vi "170519018PROJEkapalicevrimkontrolu.vi"() -> ()   [LabVIEW 2020]
uses:
  <vilib>/Instr/_visa.llb/VISA Configure Serial Port (Instr).vi
panel:
  out "ENCODER":string
  in  "PORT COM":refnum<visa-resource-name>
  in  "stop":bool
  out "PWM":i16(slide) scale=-255.0..255.0
  out "AYAR NOKTASI VE POZISYONLARI":cluster{i16, i16}(knob)={0, 73} scale=0.0..360.0
  in  "AYAR NOKTASI":i16(knob) scale=0.0..360.0
  out "GRAFIK PWM":i32(graph)
  out "GRAFIGIN AYAR NOKTASI  ve EKSEN KONUMU":cluster{"SETPOINT":i16, i32}(graph)
  # "kapali cevrim kontrolu"
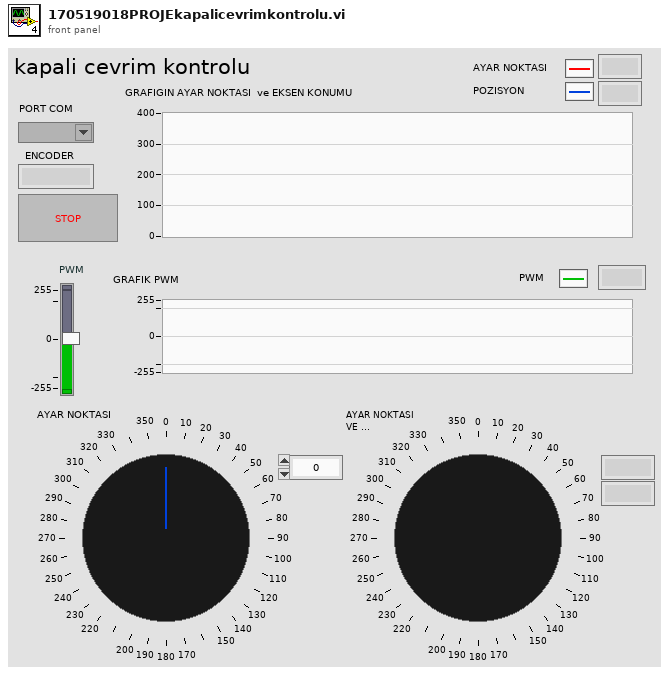
[diagram p1: front panel]
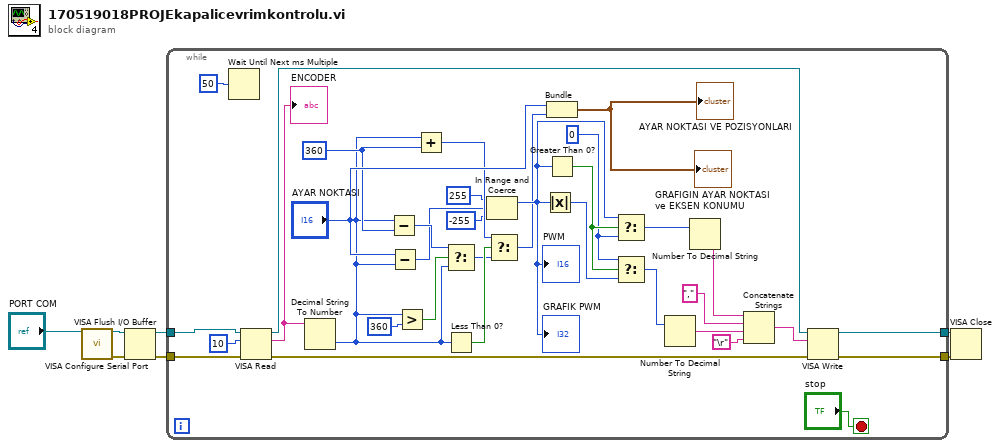
[diagram p0: block diagram]
diagram:
  n1 = call-poly "VISA Configure Serial Port"("VISA resource name"="PORT COM") -> ("VISA resource name out"=w7:refnum<visa-resource-name>, "error out"=w6:errorcluster)  [unwired: 13 in]
  n2 = VISA Flush I/O Buffer(VISA resource name=w7, error in (no error)=w6) -> (VISA resource name out=w5:refnum<visa-resource-name>, error out=w4:errorcluster)  [unwired: 1 in]
  n3 = while {
    tunnel: w5 -> [w40]
    tunnel: w4 -> [w39]
    tunnel: [w37] -> w3
    tunnel: [w36] -> w2
    stop <- "stop" stop-if-true
    w21 = 360 ("y")
    w30 = 0
    n4 = Wait Until Next ms Multiple(millisecond multiple=u32 50) -> ()  [unwired: 1 out]
    n5 = VISA Read(VISA resource name=w40, byte count=u32 10, error in (no error)=w39) -> (VISA resource name out=w41:refnum<visa-resource-name>, read buffer=w34:string, error out=w38:errorcluster)  [unwired: 1 out]
    "ENCODER" <- w34
    n6 = Decimal String To Number(string=w34) -> (number=w9:i32)  [unwired: 2 in, 1 out]
    n7 = Subtract(x=w9, y=w21) -> (x-y=w18:i32)
    n8 = Subtract(x="AYAR NOKTASI", y=w9) -> (x-y=w8:i32)
    n9 = Greater?(x=w9, y=360) -> (0:w19:bool)
    n10 = Add(x=w9, y=w21) -> (x+y=w16:i32)
    n11 = Select(t=w18, s=w19, f=w9) -> (s? t:f=w15:i32)
    n12 = Less Than 0?(x=w9) -> (x < 0?=w17:bool)
    n13 = In Range and Coerce(upper limit=255, x=w8, lower limit=-255) -> (coerced(x)=w11:i32)  [unwired: 1 out]
    "GRAFIK PWM" <- w11
    "PWM" <- w11
    n14 = Select(t=w16, s=w17, f=w15) -> (s? t:f=w10:i32)
    n15 = Absolute Value(x=w11) -> (abs(x)=w29:i32)
    n16 = Bundle("AYAR NOKTASI"="AYAR NOKTASI", w10) -> (→"GRAFIGIN AYAR NOKTASI  ve EKSEN KONUMU" →"AYAR NOKTASI VE POZISYONLARI":cluster{"AYAR NOKTASI":i16, i32})  [unwired: 1 in]
    n17 = Greater Than 0?(x=w11) -> (x > 0?=w31:bool)
    n18 = Select(t=w11, s=w31, f=w30) -> (s? t:f=w28:i32)
    n19 = Select(t=w30, s=w31, f=w29) -> (s? t:f=w27:i32)
    n20 = Number To Decimal String(number=w27) -> (decimal integer string=w24:string)  [unwired: 1 in]
    n21 = Number To Decimal String(number=w28) -> (decimal integer string=w26:string)  [unwired: 1 in]
    n22 = Concatenate Strings(w26, "," ("string"), w24, "\r") -> (w23:string)
    n23 = VISA Write(VISA resource name=w41, write buffer=w23, error in (no error)=w38) -> (VISA resource name out=w36:refnum<visa-resource-name>, error out=w37:errorcluster)  [unwired: 1 out]
  }
  n24 = VISA Close(VISA resource name=w2, error in (no error)=w3) -> ()  [unwired: 1 out]
